vi "post-reaction-test.vi"() -> ()   [LabVIEW 2023]
uses:
  <vilib>/DAQmx/read.llb/DAQmx Read (Digital 1D Bool 1Chan 1Samp).vi
  <vilib>/DAQmx/create/channels.llb/DAQmx Create Channel (DI-Digital Input).vi
  <vilib>/DAQmx/miscellaneous.llb/DAQmx Fill In Error Info.vi
panel:
  in  "V0":u16=30
  in  "V1":u16=30
  in  "index":i8
  out "sensor":bool[](array[boolean])
  in  "stop":bool
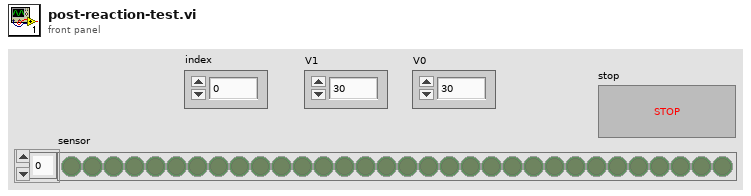
[diagram p1: front panel]
types:
  T1 = enum16{"plate1", "plate2", "plate3", "rinse", "seat"}
  T2 = enum16{"Initialize", "Absolute Position", "Relative Pickup", "Relative Dispense", "Swich valve", "Bypass"}
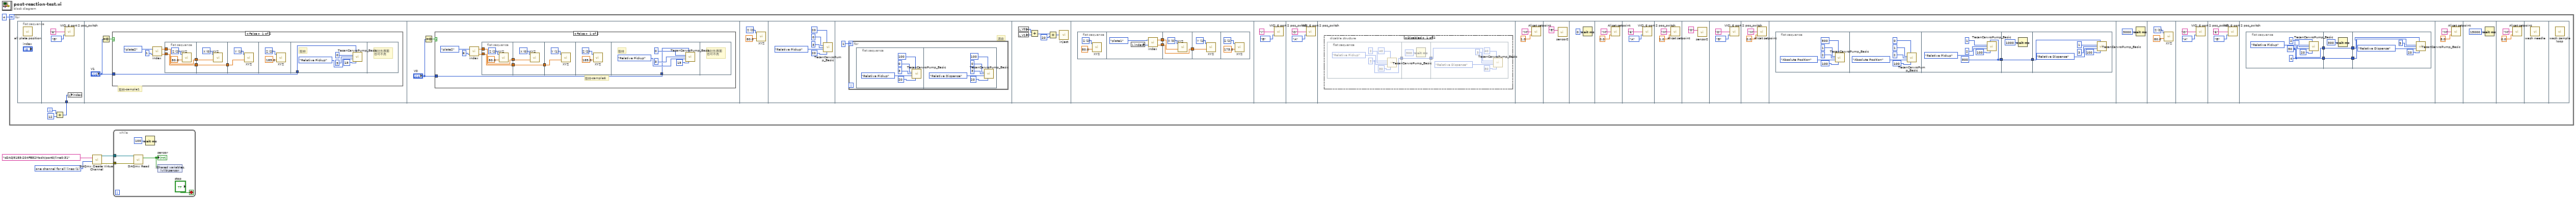
[diagram p0: block diagram]
diagram:
  w5 = 1 items=["one channel for each line", "one channel for all lines"] ("line grouping")
  n1 = for {
    N: 4 -> [_]
    i -> [w8]
    n2 = flat-sequence {
      tunnel: w6 -> [w11]
      frame #0 {
        n3 = call "all plate position.vi"() -> ()  [unwired: 3 in, 3 out]
      }
      frame #1 {
        n4 = call "VICI_6 port 2 pos_switch.vi"("Switch to position (A/B)"=enum16{"A", "B"}."B", "Valve ID"="6") -> ()  [unwired: 2 in, 1 out]
        n5 = local write "index"(w11) -> ()
      }
      frame #2 {
        # "取样-sample1"
        n6 = Equal To 0?(x="V1") -> (x = 0?=w12:bool)
        n7 = case shown="False" w12 {
          tunnel: "V1" -> [w14 _]
          frame False {
            n8 = call "index.vi"("index"=i8 1, "where"=T1."plate2") -> ("Y"=w17:dbl, "X"=w18:dbl)
            n9 = flat-sequence {
              tunnel: [w23] -> w21
              tunnel: [w22] -> w20
              tunnel: w18 -> [w23]
              tunnel: w17 -> [w22]
              tunnel: w21 -> [w27]
              tunnel: [w26] -> w19
              tunnel: w20 -> [w26]
              tunnel: w19 -> [w29]
              tunnel: w14 -> [w33]
              frame #0 {
                w25 = u16 2 items=["X", "Y", "Z"] ("AXIS")
                n10 = call "XYZ.vi"("AXIS"=w25, "Set location (mm)"=80.0) -> ()  [unwired: 9 in, 5 out]
              }
              frame #1 {
                w28 = u16 0 items=["X", "Y", "Z"] ("AXIS")
                n11 = call "XYZ.vi"("AXIS"=w28, "Set location (mm)"=w27) -> ()  [unwired: 9 in, 5 out]
              }
              frame #2 {
                w30 = u16 1 items=["X", "Y", "Z"] ("AXIS")
                n12 = call "XYZ.vi"("AXIS"=w30, "Set location (mm)"=w29) -> ()  [unwired: 9 in, 5 out]
              }
              frame #3 {
                w31 = u16 2 items=["X", "Y", "Z"] ("AXIS")
                n13 = call "XYZ.vi"("AXIS"=w31, "Set location (mm)"=185.0) -> ()  [unwired: 9 in, 5 out]
              }
              frame #4 {
                # "取样"
                n14 = call "TecanCarvroPump_Basic.vi"("Volume (μL)"=w33, "TecanPump address"=u8 0, "Valve"=u8 3, "Mode"=T2."Relative Pickup", "Speed (μL/s)"=u16 15) -> ()  [unwired: 10 in, 1 out]
              }
              frame #5 {
                # "洗针外表面\n也可不洗"
              }
            }
          }
          frame True {
          }
        }
      }
      frame #3 {
        n15 = Equal To 0?(x="V0") -> (x = 0?=w38:bool)
        n16 = case shown="False" w38 {
          tunnel: "V0" -> [w40 _]
          frame False {
            # "取样-sample6"
            n17 = call "index.vi"("index"=i8 6, "where"=T1."plate2") -> ("Y"=w42:dbl, "X"=w41:dbl)
            n18 = flat-sequence {
              tunnel: [w49] -> w47
              tunnel: [w48] -> w46
              tunnel: w41 -> [w49]
              tunnel: w42 -> [w48]
              tunnel: w47 -> [w53]
              tunnel: [w52] -> w45
              tunnel: w46 -> [w52]
              tunnel: w45 -> [w55]
              tunnel: w40 -> [w59]
              frame #0 {
                w51 = u16 2 items=["X", "Y", "Z"] ("AXIS")
                n19 = call "XYZ.vi"("AXIS"=w51, "Set location (mm)"=80.0) -> ()  [unwired: 9 in, 5 out]
              }
              frame #1 {
                w54 = u16 0 items=["X", "Y", "Z"] ("AXIS")
                n20 = call "XYZ.vi"("AXIS"=w54, "Set location (mm)"=w53) -> ()  [unwired: 9 in, 5 out]
              }
              frame #2 {
                w56 = u16 1 items=["X", "Y", "Z"] ("AXIS")
                n21 = call "XYZ.vi"("AXIS"=w56, "Set location (mm)"=w55) -> ()  [unwired: 9 in, 5 out]
              }
              frame #3 {
                w57 = u16 2 items=["X", "Y", "Z"] ("AXIS")
                n22 = call "XYZ.vi"("AXIS"=w57, "Set location (mm)"=185.0) -> ()  [unwired: 9 in, 5 out]
              }
              frame #4 {
                # "取样"
                n23 = call "TecanCarvroPump_Basic.vi"("Volume (μL)"=w59, "TecanPump address"=u8 0, "Valve"=u8 3, "Mode"=T2."Relative Pickup", "Speed (μL/s)"=u16 15) -> ()  [unwired: 10 in, 1 out]
              }
              frame #5 {
                # "洗针外表面\n也可不洗"
              }
            }
          }
          frame True {
          }
        }
      }
      frame #4 {
        w64 = u16 2 items=["X", "Y", "Z"] ("AXIS")
        n24 = call "XYZ.vi"("AXIS"=w64, "Set location (mm)"=80.0) -> ()  [unwired: 9 in, 5 out]
      }
      frame #5 {
        n25 = call "TecanCarvroPump_Basic.vi"("Volume (μL)"=u16 20, "TecanPump address"=u8 0, "Valve"=u8 3, "Mode"=T2."Relative Pickup", "Speed (μL/s)"=u16 20) -> ()  [unwired: 10 in, 1 out]
      }
      frame #6 {
        # "混合"
        n26 = for {
          N: 1 -> [_]
          n27 = flat-sequence {
            frame #0 {
              n28 = call "TecanCarvroPump_Basic.vi"("Volume (μL)"=u16 100, "TecanPump address"=u8 0, "Valve"=u8 3, "Mode"=T2."Relative Pickup", "Speed (μL/s)"=u16 20) -> ()  [unwired: 10 in, 1 out]
            }
            frame #1 {
              n29 = call "TecanCarvroPump_Basic.vi"("Volume (μL)"=u16 100, "TecanPump address"=u8 0, "Valve"=u8 3, "Mode"=T2."Relative Dispense", "Speed (μL/s)"=u16 20) -> ()  [unwired: 10 in, 1 out]
            }
          }
        }
      }
      frame #7 {
        n30 = local read "V0"() -> (w84:u16)
        n31 = local read "V1"() -> (w83:u16)
        n32 = Add(x=w84, y=w83) -> (x+y=w82:u16)
        n33 = Add(x=w82, y=20) -> (x+y=w86:i32)
        n34 = call "inject.vi"("volume"=w86) -> ()  [unwired: 1 in]
      }
      frame #8 {
        n35 = flat-sequence {
          tunnel: [w94] -> w89
          tunnel: [w93] -> w88
          tunnel: w89 -> [w96]
          tunnel: w88 -> [w98]
          tunnel: [w98] -> w87
          tunnel: w87 -> [w99]
          frame #0 {
            w90 = u16 2 items=["X", "Y", "Z"] ("AXIS")
            n36 = call "XYZ.vi"("AXIS"=w90, "Set location (mm)"=80.0) -> ()  [unwired: 9 in, 5 out]
          }
          frame #1 {
            n37 = local read "index"() -> (w92:i8)
            n38 = call "index.vi"("index"=w92, "where"=T1."plate1") -> ("Y"=w93:dbl, "X"=w94:dbl)
          }
          frame #2 {
            w97 = u16 0 items=["X", "Y", "Z"] ("AXIS")
            n39 = call "XYZ.vi"("AXIS"=w97, "Set location (mm)"=w96) -> ()  [unwired: 9 in, 5 out]
          }
          frame #3 {
            w100 = u16 1 items=["X", "Y", "Z"] ("AXIS")
            n40 = call "XYZ.vi"("AXIS"=w100, "Set location (mm)"=w99) -> ()  [unwired: 9 in, 5 out]
          }
          frame #4 {
            w102 = u16 2 items=["X", "Y", "Z"] ("AXIS")
            n41 = call "XYZ.vi"("AXIS"=w102, "Set location (mm)"=175.0) -> ()  [unwired: 9 in, 5 out]
          }
        }
      }
      frame #9 {
        n42 = call "VICI_6 port 2 pos_switch.vi"("Switch to position (A/B)"=enum16{"A", "B"}."B", "Valve ID"="I") -> ()  [unwired: 2 in, 1 out]
      }
      frame #10 {
        n43 = call "VICI_6 port 2 pos_switch.vi"("Switch to position (A/B)"=enum16{"A", "B"}."A", "Valve ID"="O") -> ()  [unwired: 2 in, 1 out]
      }
      frame #11 {
        n44 = disable-structure shown="Disabled" {
          frame Disabled {
            n45 = flat-sequence {
              tunnel: [w109] -> w108
              tunnel: w108 -> [w115]
              tunnel: [w115] -> w107
              tunnel: w107 -> [w116]
              frame #0 {
                w109 = u8 2 ("TecanPump address")
                n46 = call "TecanCarvroPump_Basic.vi"("Volume (μL)"=u16 40, "TecanPump address"=w109, "Valve"=u8 2, "Mode"=T2."Relative Pickup", "Speed (μL/s)"=u16 30) -> ()  [unwired: 10 in, 1 out]
              }
              frame #1 {
                n47 = Wait (ms)(milliseconds to wait=u32 300) -> ()  [unwired: 1 out]
              }
              frame #2 {
                n48 = call "TecanCarvroPump_Basic.vi"("Volume (μL)"=u16 40, "TecanPump address"=w116, "Valve"=u8 3, "Mode"=T2."Relative Dispense", "Speed (μL/s)"=u16 30) -> ()  [unwired: 10 in, 1 out]
              }
            }
          }
          frame Enabled {
          }
        }
      }
      frame #12 {
        n49 = call "Alicat setpoint.vi"("Setpoint"=1.0, "Unit ID"="M") -> ()  [unwired: 3 in]
      }
      frame #13 {
        n50 = call "sensor2.vi"("Sensor"="E") -> ()  [unwired: 1 in, 2 out]
      }
      frame #14 {
        n51 = Wait (ms)(milliseconds to wait=u32 0) -> ()  [unwired: 1 out]
      }
      frame #15 {
        n52 = call "Alicat setpoint.vi"("Setpoint"=0.0, "Unit ID"="M") -> ()  [unwired: 3 in]
      }
      frame #16 {
        n53 = call "VICI_6 port 2 pos_switch.vi"("Switch to position (A/B)"=enum16{"A", "B"}."A", "Valve ID"="6") -> ()  [unwired: 2 in, 1 out]
      }
      frame #17 {
        n54 = call "Alicat setpoint.vi"("Setpoint"=1.0, "Unit ID"="M") -> ()  [unwired: 3 in]
      }
      frame #18 {
        n55 = call "sensor2.vi"("Sensor"="O") -> ()  [unwired: 1 in, 2 out]
      }
      frame #19 {
        n56 = call "VICI_6 port 2 pos_switch.vi"("Switch to position (A/B)"=enum16{"A", "B"}."B", "Valve ID"="O") -> ()  [unwired: 2 in, 1 out]
      }
      frame #20 {
        n57 = call "Alicat setpoint.vi"("Setpoint"=0.0, "Unit ID"="M") -> ()  [unwired: 3 in]
      }
      frame #21 {
        n58 = flat-sequence {
          tunnel: [w148] -> w137
          tunnel: w137 -> [w154]
          tunnel: [w154] -> w136
          tunnel: w136 -> [w155]
          frame #0 {
            n59 = call "TecanCarvroPump_Basic.vi"("Volume (μL)"=u16 500, "TecanPump address"=u8 1, "Valve"=u8 2, "Mode"=T2."Absolute Position", "Speed (μL/s)"=u16 100) -> ()  [unwired: 10 in, 1 out]
          }
          frame #1 {
            n60 = call "TecanCarvroPump_Basic.vi"("Volume (μL)"=u16 0, "TecanPump address"=u8 1, "Valve"=u8 2, "Mode"=T2."Absolute Position", "Speed (μL/s)"=u16 100) -> ()  [unwired: 10 in, 1 out]
          }
          frame #2 {
            w148 = u16 500 ("Volume (μL)")
            n61 = call "TecanCarvroPump_Basic.vi"("Volume (μL)"=w148, "TecanPump address"=u8 1, "Valve"=u8 2, "Mode"=T2."Relative Pickup", "Speed (μL/s)"=u16 100) -> ()  [unwired: 10 in, 1 out]
          }
          frame #3 {
            n62 = Wait (ms)(milliseconds to wait=u32 1000) -> ()  [unwired: 1 out]
          }
          frame #4 {
            n63 = call "TecanCarvroPump_Basic.vi"("Volume (μL)"=w155, "TecanPump address"=u8 1, "Valve"=u8 3, "Mode"=T2."Relative Dispense", "Speed (μL/s)"=u16 100) -> ()  [unwired: 10 in, 1 out]
          }
        }
      }
      frame #22 {
        n64 = Wait (ms)(milliseconds to wait=u32 3000) -> ()  [unwired: 1 out]
      }
      frame #23 {
        w162 = u16 2 items=["X", "Y", "Z"] ("AXIS")
        n65 = call "XYZ.vi"("AXIS"=w162, "Set location (mm)"=80.0) -> ()  [unwired: 9 in, 5 out]
      }
      frame #24 {
        n66 = call "VICI_6 port 2 pos_switch.vi"("Switch to position (A/B)"=enum16{"A", "B"}."A", "Valve ID"="O") -> ()  [unwired: 2 in, 1 out]
      }
      frame #25 {
        n67 = call "VICI_6 port 2 pos_switch.vi"("Switch to position (A/B)"=enum16{"A", "B"}."B", "Valve ID"="6") -> ()  [unwired: 2 in, 1 out]
      }
      frame #26 {
        n68 = flat-sequence {
          tunnel: [w172] -> w170
          tunnel: [w171] -> w167
          tunnel: w170 -> [w178]
          tunnel: [w178] -> w169
          tunnel: [w176] -> w168
          tunnel: w167 -> [w176]
          tunnel: w169 -> [w180]
          tunnel: w168 -> [w179]
          frame #0 {
            w171 = u16 50 ("Volume (μL)")
            w172 = u8 4 ("TecanPump address")
            n69 = call "TecanCarvroPump_Basic.vi"("Volume (μL)"=w171, "TecanPump address"=w172, "Valve"=u8 2, "Mode"=T2."Relative Pickup", "Speed (μL/s)"=u16 20) -> ()  [unwired: 10 in, 1 out]
          }
          frame #1 {
            n70 = Wait (ms)(milliseconds to wait=u32 300) -> ()  [unwired: 1 out]
          }
          frame #2 {
            n71 = call "TecanCarvroPump_Basic.vi"("Volume (μL)"=w179, "TecanPump address"=w180, "Valve"=u8 3, "Mode"=T2."Relative Dispense", "Speed (μL/s)"=u16 20) -> ()  [unwired: 10 in, 1 out]
          }
        }
      }
      frame #27 {
        n72 = call "Alicat setpoint.vi"("Setpoint"=8.0, "Unit ID"="M") -> ()  [unwired: 3 in]
      }
      frame #28 {
        n73 = Wait (ms)(milliseconds to wait=u32 15000) -> ()  [unwired: 1 out]
      }
      frame #29 {
        n74 = call "Alicat setpoint.vi"("Setpoint"=0.0, "Unit ID"="M") -> ()  [unwired: 3 in]
      }
      frame #30 {
        n75 = call "wash needle.vi"() -> ()  [unwired: 12 in]
      }
      frame #31 {
        n76 = call "wash sample loop.vi"() -> ()  [unwired: 12 in]
      }
    }
    n77 = Add(x=w8, y=12) -> (x+y=w6:i32)
  }
  n78 = call-poly <vilib>:"DAQmx Create Virtual Channel.vi"("lines"=tag "cDAQ9185-204FB52Mod4/port0/line0:31", "line grouping"=w5) -> ("task out"=w4:refnum<k21>, "error out"=w3:errorcluster)  [unwired: 12 in]
  n79 = while {
    tunnel: w4 -> [w193]
    tunnel: w3 -> [w192]
    stop <- "stop" stop-if-true
    n80 = call-poly <vilib>:"DAQmx Read.vi"("task/channels in"=w193, "error in"=w192) -> ("data"=w191:bool[])  [unwired: 11 in, 2 out]
    "sensor" <- w191
    n81 = Wait (ms)(milliseconds to wait=u32 100) -> ()  [unwired: 1 out]
    n82 = shared-variable ".\\Shared variables.lvlib\\sensor"(w191) -> ()  [unwired: 1 in, 1 out]
  }
